vi "Agua.vi"(8 "error in (no error)":errorcluster, 11 "Productos in":refnum<class "Productos.lvclass">) -> (0 "error out":errorcluster, 3 "Productos out":refnum<class "Productos.lvclass">)   [LabVIEW 2020, in "Productos.lvlib" / "Productos.lvclass"]
uses:
  Productos.lvclass
  C:/Program Files (x86)/National Instruments/LabVIEW 2020/vi.lib/ActorFramework/Actor/Actor.lvclass
  <vilib>/ActorFramework/Actor/Actor.lvclass/Actor.ctl
  <vilib>/ActorFramework/Message Enqueuer/Message Enqueuer.lvclass/Message Enqueuer.ctl
  Productos.lvclass/Productos.ctl
  User Interface Messages/Productos Msg/Productos Msg.lvclass/Productos Msg.ctl
  Productos Messages/Write agua Inv Msg/Write agua Inv Msg.lvclass/Write agua Inv Msg.ctl
  <vilib>/ActorFramework/Message Enqueuer/Init from Existing Queue.vi
  <vilib>/ActorFramework/Message Enqueuer/Enqueue.vi
  User Interface Messages/Productos Msg/Productos Msg.lvclass
  C:/Program Files (x86)/National Instruments/LabVIEW 2020/vi.lib/ActorFramework/Message/Message.lvclass
  Productos Messages/Write agua Inv Msg/Write agua Inv Msg.lvclass
  Productos Messages/Read Inventory Msg/Read Inventory Msg.lvclass
  <vilib>/ActorFramework/Message Priority Queue/Priority Enqueue.vi
  <vilib>/ActorFramework/Message Enqueuer/Message Enqueuer.lvclass
  <vilib>/ActorFramework/Actor/Actor.lvclass
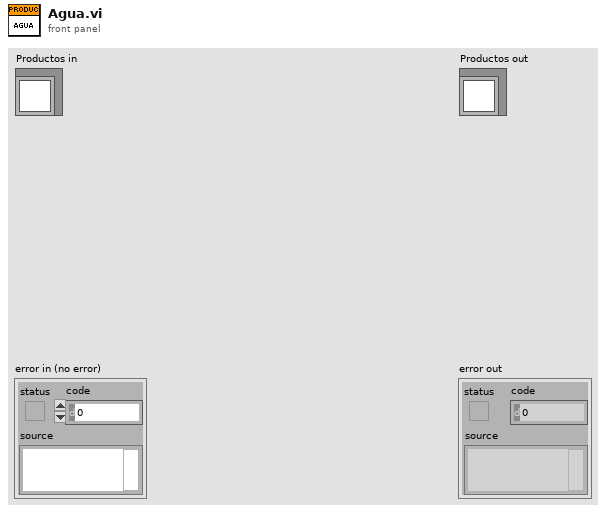
[diagram p1: front panel]
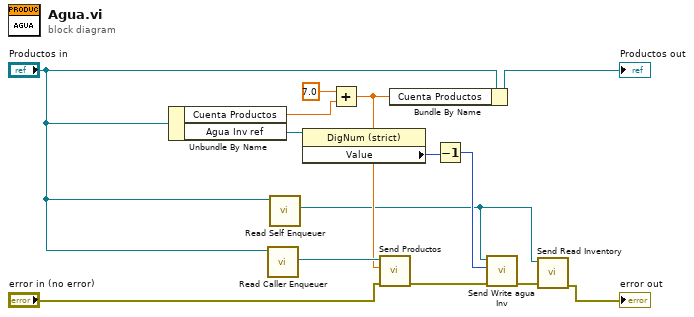
[diagram p0: block diagram]
diagram:
  n1 = Unbundle By Name("Productos in") -> ("Cuenta Productos"=w14:dbl, "Agua Inv ref"=w4:refnum<vi>)
  n2 = call <vilib>:"Read Caller Enqueuer.vi"("Actor"="Productos in") -> ("Caller Enqueuer"=w10:refnum<class "Message Enqueuer.lvclass">)  [unwired: 10 in]
  n3 = call <vilib>:"Read Self Enqueuer.vi"("Actor"="Productos in") -> ("Self Enqueuer"=w1:refnum<class "Message Enqueuer.lvclass">)  [unwired: 10 in]
  n4 = property class="DigNum (strict)"(reference=w4) -> ("Value"=w3:i32)  [unwired: 1 in, 2 out]
  n5 = Add(x=7.0, y=w14) -> (x+y=w9:dbl)
  n6 = call "Send Productos.vi"("error in (no error)"="error in (no error)", "Productos"=w9, "Message Enqueuer"=w10) -> ("error out"=w6:errorcluster)  [unwired: 7 in, 1 out]
  n7 = Bundle By Name(cluster="Productos in", "Cuenta Productos"=w9) -> (→"Productos out":refnum<class "Productos.lvclass">)
  n8 = Decrement(x=w3) -> (x-1=w2:i32)
  n9 = call "Send Write agua Inv.vi"("error in (no error)"=w6, "Agua"=w2, "Message Enqueuer"=w1) -> ("error out"=w7:errorcluster)  [unwired: 7 in, 1 out]
  n10 = call "Send Read Inventory.vi"("error in (no error)"=w7, "Message Enqueuer"=w1) -> ("error out"=→"error out":errorcluster)  [unwired: 8 in, 1 out]
